vi "Write GameRef.vi"(8 "error in (no error)":errorcluster, 10 "GameRef":refnum<data-value>, 11 "PassObjective in":refnum<class "PassObjective.lvclass">) -> (0 "error out":errorcluster, 3 "PassObjective out":refnum<class "PassObjective.lvclass">)   [LabVIEW 2023, in "PassObjective.lvclass"]
uses:
  PassObjective.lvclass
  Game_class/Game.lvclass
  PassObjective.lvclass/PassObjective.ctl
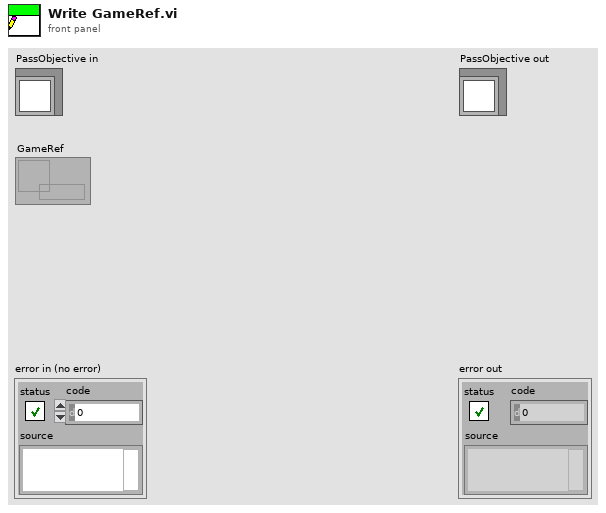
[diagram p1: front panel]
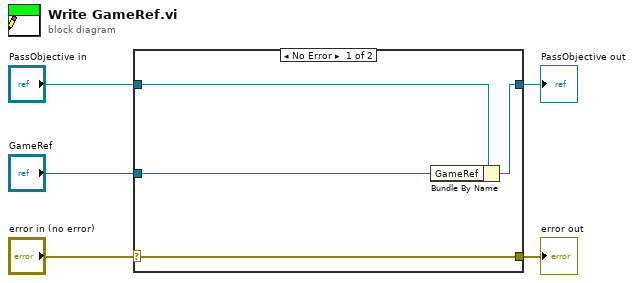
[diagram p0: block diagram]
diagram:
  n1 = case shown="No Error" "error in (no error)" {
    selector: "error in (no error)" -> [w9 w10]
    tunnel: [w9 w10] -> w4
    tunnel: [w7 w11] -> w2
    tunnel: "PassObjective in" -> [w8 w11]
    tunnel: "GameRef" -> [w6 _]
    frame No Error {
      n2 = Bundle By Name(cluster=w8, "GameRef"=w6) -> (w7:refnum<class "PassObjective.lvclass">)
    }
    frame Error {
    }
  }
  "error out" <- w4
  "PassObjective out" <- w2
